vi "Make Color Table.vi"(0 "Array":u32[](array[colorbox]), 1 "Size/3":i32=256) -> (2 "Array R":dbl[](array[numeric]), 3 "Array G":dbl[](array[numeric]), 4 "Array B":dbl[](array[numeric]), 5 "Color Tbl":u32[](array[numeric]))   [LabVIEW 2016]
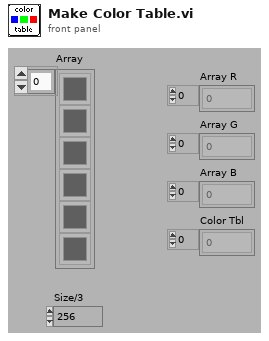
[diagram p1: front panel]
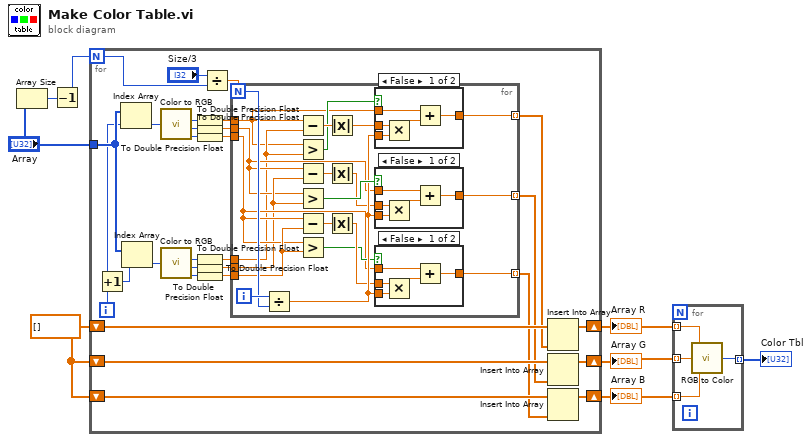
[diagram p0: block diagram]
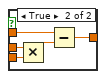
[diagram p2: hidden frame]
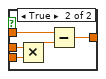
[diagram p3: hidden frame]
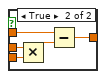
[diagram p4: hidden frame]
diagram:
  w5 = dbl[] []
  n1 = Array Size(array="Array") -> (size(s)=w8:i32)
  n2 = Decrement(x=w8) -> (x-1=w7:i32)
  n3 = for {
    N: w7 -> [w10]
    tunnel: "Array" -> [w36]
    shift-right: [w32] -> w4
    shift-left: w5 -> [w17]
    shift-right: [w31] -> w3
    shift-left: w5 -> [w16]
    shift-right: [w30] -> w2
    shift-left: w5 -> [w15]
    i -> [w33]
    n4 = Increment(x=w33) -> (x+1=w34:i32)
    n5 = Index Array(array=w36, index=w33) -> (element=w35:u32)
    n6 = Index Array(array=w36, index=w34) -> (element=w37:u32)
    n7 = call <vilib>:"Color to RGB.vi"("Color"=w35) -> ("R"=w29:u8, "G"=w28:u8, "B"=w27:u8)  [unwired: 1 out]
    n8 = call <vilib>:"Color to RGB.vi"("Color"=w37) -> ("R"=w26:u8, "G"=w25:u8, "B"=w24:u8)  [unwired: 1 out]
    n9 = To Double Precision Float(number=w29) -> (double precision float=w23:dbl)
    n10 = To Double Precision Float(number=w28) -> (double precision float=w22:dbl)
    n11 = To Double Precision Float(number=w27) -> (double precision float=w21:dbl)
    n12 = To Double Precision Float(number=w26) -> (double precision float=w20:dbl)
    n13 = To Double Precision Float(number=w25) -> (double precision float=w19:dbl)
    n14 = To Double Precision Float(number=w24) -> (double precision float=w18:dbl)
    n15 = Divide(x="Size/3", y=w10) -> (x/y=w9:dbl)
    n16 = for {
      N: w9 -> [w52]
      tunnel: w23 -> [w38]
      tunnel: w20 -> [w39]
      tunnel: w19 -> [w41]
      tunnel: w18 -> [w43]
      tunnel: w22 -> [w40]
      tunnel: w21 -> [w42]
      tunnel: [w51] -> w12 mode=indexing
      tunnel: [w45] -> w13 mode=indexing
      tunnel: [w44] -> w14 mode=indexing
      i -> [w53]
      n17 = Divide(x=w53, y=w52) -> (x/y=w49:dbl)
      n18 = Subtract(x=w38, y=w39) -> (x-y=w58:dbl)
      n19 = Greater?(x=w38, y=w39) -> (0:w55:bool)
      n20 = Subtract(x=w40, y=w41) -> (x-y=w57:dbl)
      n21 = Greater?(x=w40, y=w41) -> (0:w50:bool)
      n22 = Subtract(x=w42, y=w43) -> (x-y=w56:dbl)
      n23 = Greater?(x=w42, y=w43) -> (0:w46:bool)
      n24 = Absolute Value(x=w58) -> (abs(x)=w54:dbl)
      n25 = Absolute Value(x=w57) -> (abs(x)=w47:dbl)
      n26 = Absolute Value(x=w56) -> (abs(x)=w48:dbl)
      n27 = case shown="False" w55 {
        tunnel: w54 -> [w81 w88]
        tunnel: w38 -> [w80 w85]
        tunnel: w49 -> [w82 w87]
        tunnel: [w79 w84] -> w51
        frame False {
          n28 = Multiply(x=w81, y=w82) -> (x*y=w83:dbl)
          n29 = Add(x=w80, y=w83) -> (x+y=w79:dbl)
        }
        frame True {
          n30 = Multiply(x=w88, y=w87) -> (x*y=w86:dbl)
          n31 = Subtract(x=w85, y=w86) -> (x-y=w84:dbl)
        }
      }
      n32 = case shown="False" w50 {
        tunnel: w47 -> [w71 w78]
        tunnel: w40 -> [w70 w75]
        tunnel: w49 -> [w72 w77]
        tunnel: [w69 w74] -> w45
        frame False {
          n33 = Multiply(x=w71, y=w72) -> (x*y=w73:dbl)
          n34 = Add(x=w70, y=w73) -> (x+y=w69:dbl)
        }
        frame True {
          n35 = Multiply(x=w78, y=w77) -> (x*y=w76:dbl)
          n36 = Subtract(x=w75, y=w76) -> (x-y=w74:dbl)
        }
      }
      n37 = case shown="False" w46 {
        tunnel: w48 -> [w61 w68]
        tunnel: w42 -> [w60 w65]
        tunnel: w49 -> [w62 w67]
        tunnel: [w59 w64] -> w44
        frame False {
          n38 = Multiply(x=w61, y=w62) -> (x*y=w63:dbl)
          n39 = Add(x=w60, y=w63) -> (x+y=w59:dbl)
        }
        frame True {
          n40 = Multiply(x=w68, y=w67) -> (x*y=w66:dbl)
          n41 = Subtract(x=w65, y=w66) -> (x-y=w64:dbl)
        }
      }
    }
    n42 = Insert Into Array(array=w17, new element=w12) -> (w32:dbl[])  [unwired: 1 in]
    n43 = Insert Into Array(array=w16, new element=w13) -> (w31:dbl[])  [unwired: 1 in]
    n44 = Insert Into Array(array=w15, new element=w14) -> (w30:dbl[])  [unwired: 1 in]
  }
  "Array R" <- w4
  "Array G" <- w3
  "Array B" <- w2
  n45 = for {
    tunnel: w4 -> [w92] mode=indexing
    tunnel: w3 -> [w91] mode=indexing
    tunnel: w2 -> [w90] mode=indexing
    tunnel: [w89] -> w1 mode=indexing
    n46 = call <vilib>:"RGB to Color.vi"("B"=w90, "G"=w91, "R"=w92) -> ("Color"=w89:u32)
  }
  "Color Tbl" <- w1
